vi "Add Function.vi"(8 "x":dbl) -> (3 "x+y":dbl)   [LabVIEW 2018]
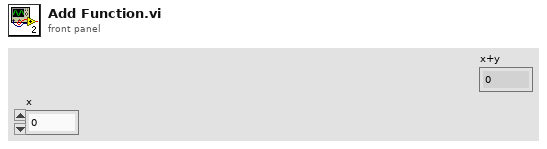
[diagram p1: front panel]
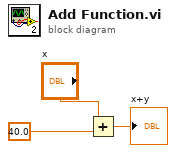
[diagram p0: block diagram]
diagram:
  n1 = Add(x="x", y=40.0) -> (x+y=→"x+y":dbl)
